vi "PAS_set_regulation_range.vi"(8 "error in (no error)":errorcluster, 9 "Range B":bool, 10 "Range A":bool, 11 "VISA Refnum in":refnum<visa-resource-name>) -> (0 "error out":errorcluster, 1 "Success?":bool, 3 "VISA Refnum out":refnum<visa-resource-name>)   [LabVIEW 2020]
panel:
  out "length":i32
  out "read buffer":string
  out "decimal integer string":string
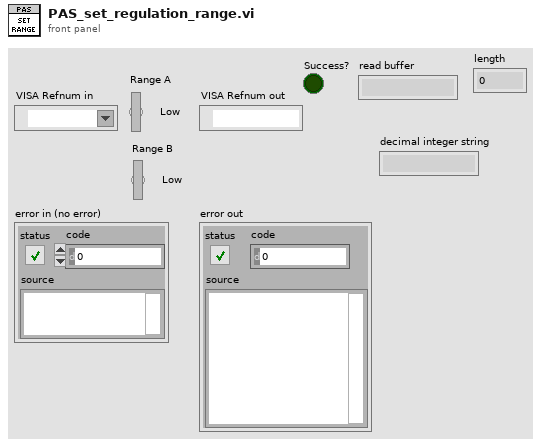
[diagram p1: front panel]
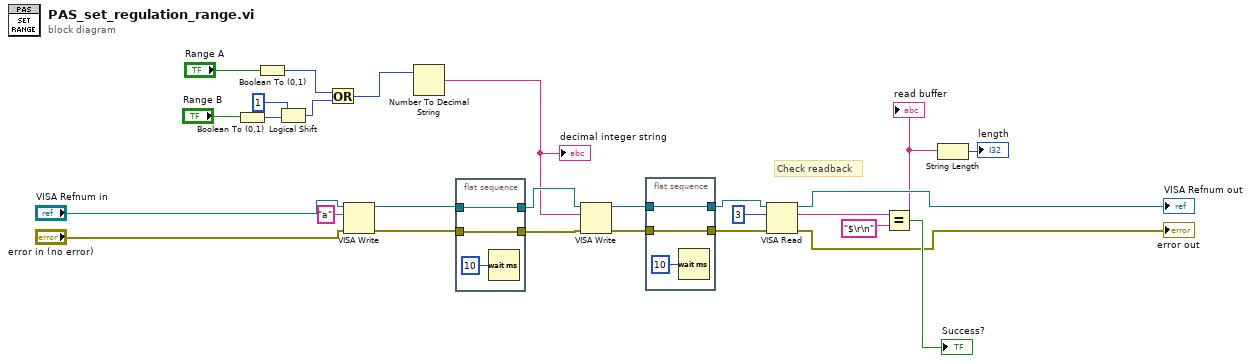
[diagram p0: block diagram]
diagram:
  # "Check readback"
  n1 = Boolean To (0,1)(Boolean="Range B") -> (0, 1=w13:i16)
  n2 = Boolean To (0,1)(Boolean="Range A") -> (0, 1=w10:i16)
  n3 = Logical Shift(y=i16 1, x=w13) -> (x << y=w11:i16)
  n4 = Or(x=w10, y=w11) -> (x .or. y?=w9:i16)
  n5 = VISA Write(VISA resource name="VISA Refnum in", write buffer="a", error in (no error)="error in (no error)") -> (VISA resource name out=w21:refnum<visa-resource-name>, error out=w22:errorcluster)  [unwired: 1 out]
  n6 = Number To Decimal String(number=w9) -> (decimal integer string=w19:string)  [unwired: 1 in]
  "decimal integer string" <- w19
  n7 = flat-sequence {
    tunnel: w21 -> [w28]
    tunnel: [w28] -> w23
    tunnel: w22 -> [w27]
    tunnel: [w27] -> w24
    frame #0 {
      n8 = Wait (ms)(milliseconds to wait=u32 10) -> ()  [unwired: 1 out]
    }
  }
  n9 = VISA Write(VISA resource name=w23, write buffer=w19, error in (no error)=w24) -> (VISA resource name out=w2:refnum<visa-resource-name>, error out=w4:errorcluster)  [unwired: 1 out]
  n10 = flat-sequence {
    tunnel: w2 -> [w31]
    tunnel: [w31] -> w1
    tunnel: w4 -> [w30]
    tunnel: [w30] -> w3
    frame #0 {
      n11 = Wait (ms)(milliseconds to wait=u32 10) -> ()  [unwired: 1 out]
    }
  }
  n12 = VISA Read(VISA resource name=w1, byte count=u32 3, error in (no error)=w3) -> (VISA resource name out=→"VISA Refnum out":refnum<visa-resource-name>, read buffer=w8:string, error out=→"error out":errorcluster)  [unwired: 1 out]
  "read buffer" <- w8
  n13 = Equal?(x=w8, y="$\r\n") -> (x = y?=→"Success?":bool)
  n14 = String Length(string=w8) -> (length=→"length":i32)
